vi "NML data acq file name number.vi"(11 "String in":string) -> (3 "String out":string)   [LabVIEW 2019]
panel:
  # "Extract numbering info from the \nNML Data Acq created data file.\nWorks for old data acq.vi  (no extention) or new  version (.txt or .text extension)"
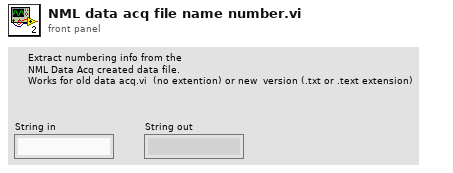
[diagram p1: front panel]
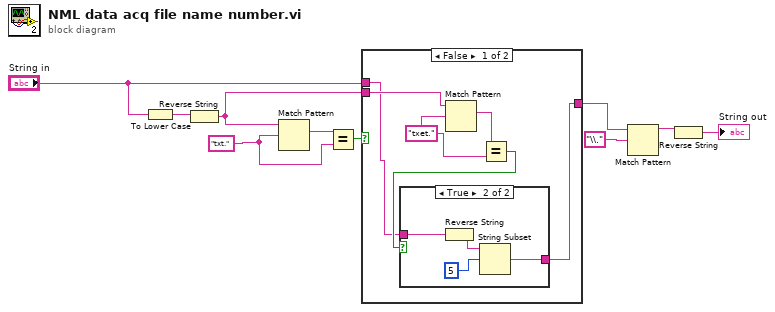
[diagram p0: block diagram]
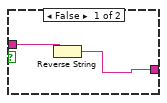
[diagram p2: hidden frame]
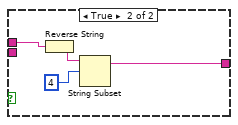
[diagram p3: hidden frame]
diagram:
  w3 = "txt." ("regular expression")
  n1 = To Lower Case(string="String in") -> (all lower case string=w1:string)
  n2 = Reverse String(1:w1) -> (0:w9:string)
  n3 = Match Pattern(string=w9, regular expression=w3) -> (match substring=w2:string)  [unwired: 1 in, 3 out]
  n4 = Equal?(x=w2, y=w3) -> (x = y?=w4:bool)
  n5 = case shown="False" w4 {
    tunnel: "String in" -> [w11 w26]
    tunnel: [w12 w23] -> w5
    tunnel: w9 -> [w16 _]
    frame False {
      w14 = "txet." ("regular expression")
      n6 = Match Pattern(string=w16, regular expression=w14) -> (match substring=w15:string)  [unwired: 1 in, 3 out]
      n7 = Equal?(x=w15, y=w14) -> (x = y?=w13:bool)
      n8 = case shown="True" w13 {
        tunnel: w11 -> [w18 w20]
        tunnel: [w17 w19] -> w12
        frame False {
          n9 = Reverse String(1:w18) -> (0:w17:string)
        }
        frame True {
          n10 = Reverse String(1:w20) -> (0:w22:string)
          n11 = String Subset(string=w22, offset (0)=5) -> (substring=w19:string)  [unwired: 1 in]
        }
      }
    }
    frame True {
      n12 = Reverse String(1:w26) -> (0:w25:string)
      n13 = String Subset(string=w25, offset (0)=4) -> (substring=w23:string)  [unwired: 1 in]
    }
  }
  n14 = Match Pattern(string=w5, regular expression="\\.") -> (before substring=w7:string)  [unwired: 1 in, 3 out]
  n15 = Reverse String(1:w7) -> (0:→"String out":string)
